vi "rate_limit_single.vi"(9 "Sample Period":dbl=0.01, 10 "Rate Limit":dbl=0.01, 11 "Input":dbl=0.01) -> (3 "Output":dbl)   [LabVIEW 2014]
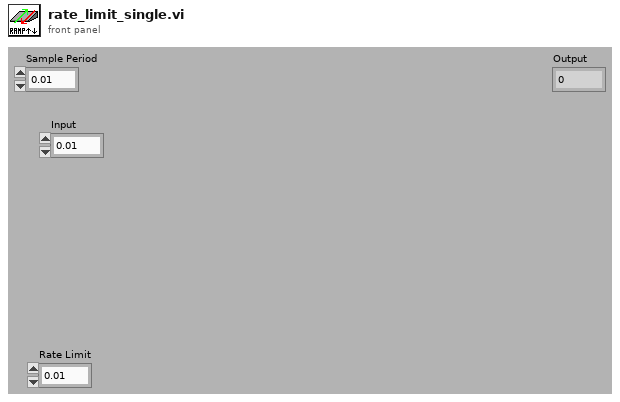
[diagram p1: front panel]
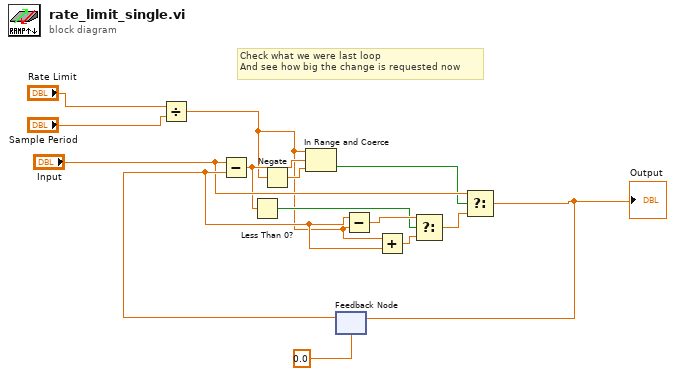
[diagram p0: block diagram]
diagram:
  # "Check what we were last loop\nAnd see how big the change is requested now"
  n1 = Divide(x="Rate Limit", y="Sample Period") -> (x/y=w1:dbl)
  n2 = Negate(x=w1) -> (-x=w11:dbl)
  n3 = feedback #1(0.0 ("Signal")) -> (w14:dbl)
  n4 = Subtract(x="Input", y=w14) -> (x-y=w9:dbl)
  n5 = Less Than 0?(x=w9) -> (x < 0?=w6:bool)
  n6 = In Range and Coerce(upper limit=w1, x=w9, lower limit=w11) -> (In Range?=w5:bool)  [unwired: 1 out]
  n7 = Subtract(x=w14, y=w1) -> (x-y=w8:dbl)
  n8 = Add(x=w1, y=w14) -> (x+y=w7:dbl)
  n9 = Select(t=w8, s=w6, f=w7) -> (s? t:f=w10:dbl)
  n10 = Select(t="Input", s=w5, f=w10) -> (s? t:f=w13:dbl)
  "Output" <- w13
  n11 = feedback-in #1(w13) -> ()
